vi "Digital Write.vi"(8 "Error In":errorcluster, 10 "Digital Values":T1[](array[typedef]), 11 "LINX Resource":T2) -> (0 "Error Out":errorcluster, 3 "LINX Resource":T2)   [LabVIEW 2011, in "LVH-LINX.lvlib"]
doc: "Write the specified values on the selected digital output pins."
uses:
  <vilib>/LabVIEW Hacker/LINX/LVH-LINX.lvlib
  Private/Type Defs/LINX Ref.ctl
  Private/Type Defs/Platform.ctl
  Private/Type Defs/Interface.ctl
  Private/Device/Type Defs/LINX Device Config.ctl
  Private/Device/Type Defs/TCP Config.ctl
  Private/Type Defs/Device Family.ctl
  Private/Type Defs/Peripherals/Digital/Digital Write Control.ctl
  Private/Type Defs/Peripheral.ctl
  <vilib>/LabVIEW Hacker/LINX/Private/Device/Device.lvlib
  <vilib>/LabVIEW Hacker/LINX/Private/myRIO/myRIO.lvlib
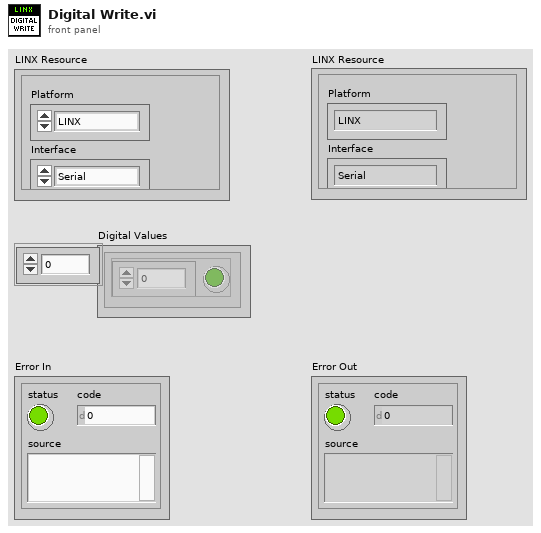
[diagram p1: front panel]
types:
  T1 = typedef "LVH-LINX.lvlib/Digital Write Control.ctl" = cluster{"Pin Number":u8, "Value":bool}
  T2 = typedef "LVH-LINX.lvlib/LINX Ref.ctl" = cluster{"Platform":T3, "Interface":T4, "LINX Device Config":T5}
  T3 = typedef "LVH-LINX.lvlib/Platform.ctl" = enum16{"LINX", "myRIO"}
  T4 = typedef "LVH-LINX.lvlib/Interface.ctl" = enum16{"Serial", "TCP"}
  T5 = typedef "LVH-LINX.lvlib/Device.lvlib/LINX Device Config.ctl" = cluster{"Interface":T4, "COM Port":refnum<visa-resource-name>, "TCP Configuration":T6, "Device ID":u8, "Device Name":string, "Device Family":T7}
  T6 = typedef "LVH-LINX.lvlib/Device.lvlib/TCP Config.ctl" = cluster{"IP Address":string, "Port":dbl}
  T7 = typedef "LVH-LINX.lvlib/Device Family.ctl" = enum8{"National Instruments", "Digilent", "Arduino"}
  T8 = typedef "LVH-LINX.lvlib/Peripheral.ctl" = enum8{"DI", "DO", "AI", "AO", "PWM", "QE", "UART", "I2C", "SPI", "CAN"}
  T9 = typedef "DIO.lvlib/DIO Reference.ctl" = cluster{"myRIO Reference":T10, "DIO Channels List":T14}
  T10 = typedef "myRIO Generic Hardware Reference.ctl" = cluster{"myRIO Model":T11, "myRIO Hardware Reference":T12}
  T11 = typedef "Hardware Version Enum.ctl" = enum16{"Unknown", "myRIO-1900", "myRIO-1950"}
  T12 = typedef "myRIO v1.0 Reference.ctl" = cluster{"Generic FPGA Reference":T13, "Allow multiple opens":bool}
  T13 = typedef "Generic FPGA Reference.ctl" = refnum<k20>
  T14 = typedef "DIO Channels List.ctl" = T15[]
  T15 = typedef "DIO Channels Enum.ctl" = enum16{"Not Connected", "C/DIO0", "C/DIO1", "C/DIO2", "C/DIO3", "C/DIO4", "C/DIO5", "C/DIO6", "C/DIO7", "A/DIO0", "A/DIO1", "A/DIO2", "A/DIO3", "A/DIO4", "A/DIO5", "A/DIO6", "A/DIO7", "A/DIO8", "A/DIO9", "A/DIO10", "A/DIO11", "A/DIO12", "A/DIO13", "A/DIO14", "A/DIO15", "B/DIO0", "B/DIO1", "B/DIO2", "B/DIO3", "B/DIO4", "B/DIO5", "B/DIO6", "B/DIO7", "B/DIO8", "B/DIO9", "B/DIO10", "B/DIO11", "B/DIO12", "B/DIO13", "B/DIO14", "B/DIO15", "LED0", "LED1", "LED2", "LED3", "Button0"}
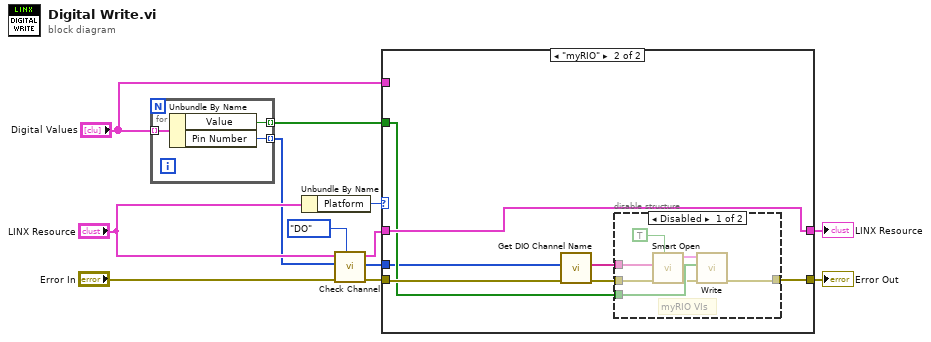
[diagram p0: block diagram]
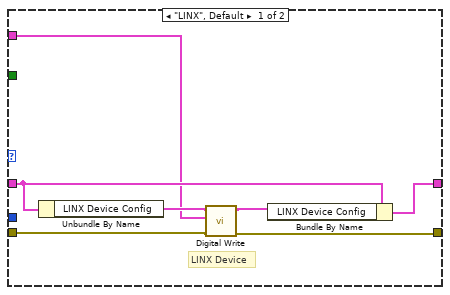
[diagram p2: hidden frame]
diagram:
  n1 = for {
    tunnel: "Digital Values" -> [w15] mode=indexing
    tunnel: [w14] -> w1 mode=indexing
    tunnel: [w13] -> w2 mode=indexing
    n2 = Unbundle By Name(w15) -> ("Value"=w14:bool, "Pin Number"=w13:u8)
  }
  n3 = Unbundle By Name("LINX Resource") -> ("Platform"=w12:T3)
  n4 = call "Check Channel.vi"("Peripheral"=Peripheral."DO", "Error In"="Error In", "Channels"=w2, "LINX Resource"="LINX Resource") -> ("Error Out"=w5:errorcluster, "Channels"=w3:u8[], "LINX Resource"=w7:T2)  [unwired: 5 in]
  n5 = case shown="\"myRIO\"" w12 {
    tunnel: w5 -> [w16 w28]
    tunnel: w7 -> [w22 w29]
    tunnel: [w20 w25] -> w11
    tunnel: [w21 w29] -> w10
    tunnel: "Digital Values" -> [w17 _]
    tunnel: w1 -> [_ w24]
    tunnel: w3 -> [_ w23]
    frame "LINX", Default {
      # "LINX Device"
      n6 = Unbundle By Name(w22) -> ("LINX Device Config"=w18:T5)
      n7 = call "Digital Write.vi"("Error In"=w16, "Digital Values"=w17, "LINX Device Config"=w18) -> ("Error Out"=w20:errorcluster, "LINX Device Config"=w19:T5)  [unwired: 7 in]
      n8 = Bundle By Name(cluster=w22, "LINX Device Config"=w19) -> (w21:T2)
    }
    frame "myRIO" {
      n9 = call "Get DIO Channel Name.vi"("Error In"=w28, "DIO Channel Nums"=w23) -> ("Error Out"=w26:errorcluster, "DIO Channels"=w27:string[])  [unwired: 8 in]
      n10 = disable-structure shown="Disabled" {
        disable-tunnel: w27 -> [w32 _]
        disable-tunnel: w26 -> [w33 w37]
        disable-tunnel: w24 -> [w36 _]
        disable-tunnel: [w35 w37] -> w25
        frame Disabled {
          # "myRIO VIs"
          n11 = call <vilib>:"Smart Open.vi"("Allow multiple opens?"=TRUE, "error in (no error)"=w33, "Channel Names"=w32) -> ("error out"=w34:errorcluster, "DIO Ref Out"=w31:T9)  [unwired: 7 in]
          n12 = call <vilib>:"Write.vi"("error in (no error)"=w34, "Values"=w36, "DIO Ref In"=w31) -> ("error out"=w35:errorcluster)  [unwired: 6 in, 1 out]
        }
        frame Enabled {
          # "myRIO Support Disabled"
        }
      }
    }
  }
  "Error Out" <- w11
  "LINX Resource" <- w10
